vi "Select Alarm.vi"(8 "error in (no error)":errorcluster, 10 "Alarm":u16(ring) items=["A", "B", "C", "D"], 11 "VISA resource name":refnum<visa-resource-name>) -> (0 "error out":errorcluster, 3 "VISA resource name out":refnum<visa-resource-name>)   [LabVIEW 2017, in "Sefram DAS220.lvlib"]
uses:
  <instrlib>/Sefram DAS220/Sefram DAS220.lvlib
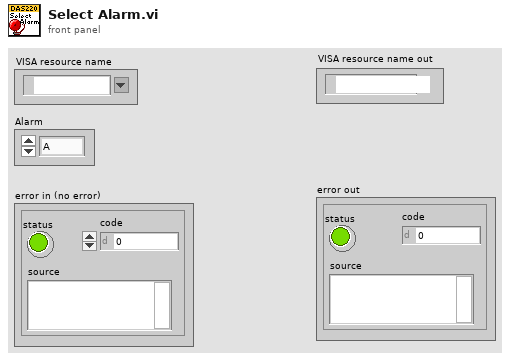
[diagram p1: front panel]
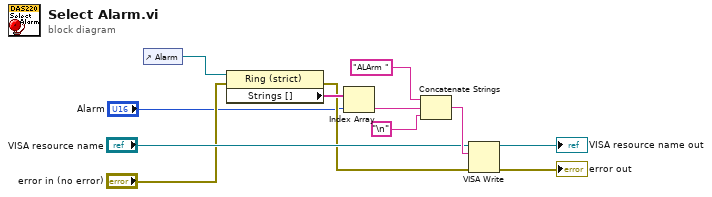
[diagram p0: block diagram]
diagram:
  n1 = control-ref of="Alarm"() -> (w1:refnum<vi>)
  n2 = property class="Ring (strict)"(reference=w1, error in="error in (no error)") -> (error out=w3:errorcluster, "Strings []"=w8:string[])  [unwired: 1 out]
  n3 = Index Array(array=w8, index="Alarm") -> (element=w7:string)
  n4 = Concatenate Strings("ALArm " ("string"), w7, "\n") -> (w11:string)
  n5 = VISA Write(VISA resource name="VISA resource name", write buffer=w11, error in (no error)=w3) -> (VISA resource name out=→"VISA resource name out":refnum<visa-resource-name>, error out=→"error out":errorcluster)  [unwired: 1 out]
